vi "Read Writing Setpoint.vi"(8 "error in (no error)":errorcluster, 11 "AFM_Driver in":refnum<class "AFM_Driver.lvclass">) -> (0 "error out":errorcluster, 2 "Writing Setpoint":dbl=0.1 format="%#_13g", 3 "AFM_Driver out":refnum<class "AFM_Driver.lvclass">)   [LabVIEW 2019, in "AFM_Driver.lvclass"]
uses:
  AFM_Driver.lvclass
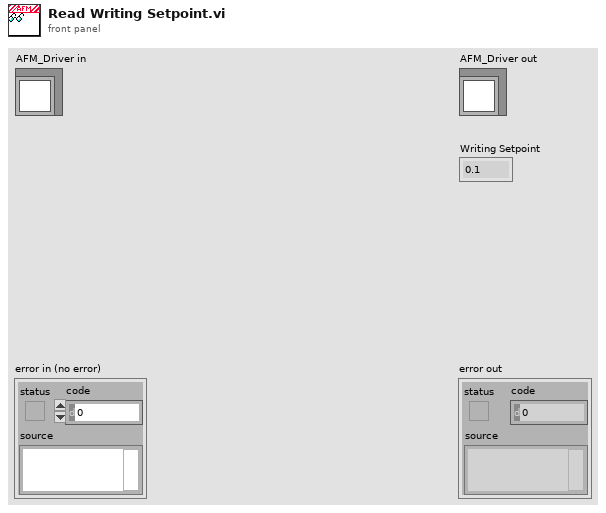
[diagram p1: front panel]
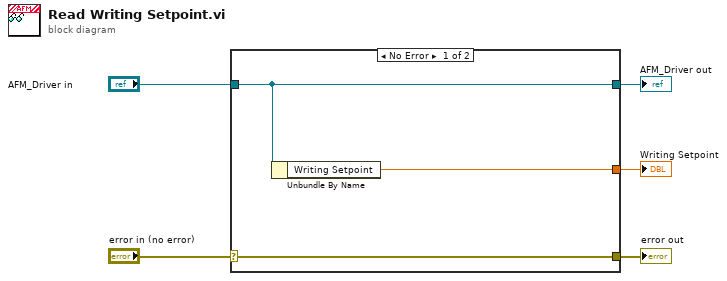
[diagram p0: block diagram]
diagram:
  n1 = case shown="No Error" "error in (no error)" {
    selector: "error in (no error)" -> [w8 w9]
    tunnel: [w8 w9] -> w4
    tunnel: [w7 w10] -> w2
    tunnel: "AFM_Driver in" -> [w7 w10]
    tunnel: [w6 _] -> w1
    frame No Error {
      n2 = Unbundle By Name(w7) -> ("Writing Setpoint"=w6:dbl)
    }
    frame Error {
    }
  }
  "error out" <- w4
  "AFM_Driver out" <- w2
  "Writing Setpoint" <- w1
